vi "Read Dialog Text.vi"(8 "error in (no error)":errorcluster, 11 "Dialog in":refnum<class "Dialog.lvclass">) -> (0 "error out":errorcluster, 2 "Dialog Text":string, 3 "Dialog out":refnum<class "Dialog.lvclass">)   [LabVIEW 2020, in "Dialog Classes.lvlib" / "Dialog.lvclass"]
uses:
  Dialog.lvclass
  Dialog.lvclass/Dialog.ctl
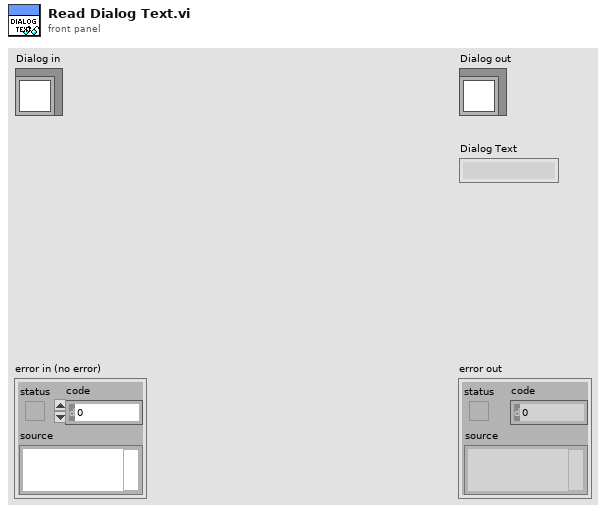
[diagram p1: front panel]
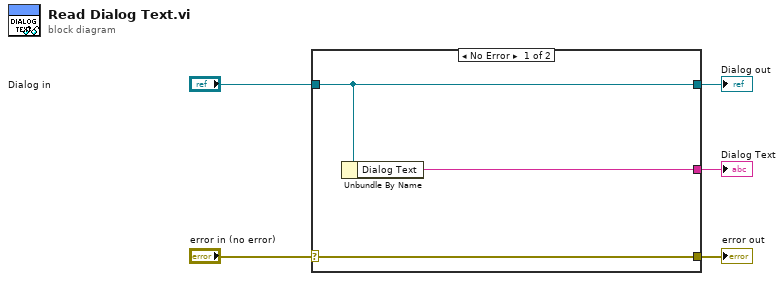
[diagram p0: block diagram]
diagram:
  n1 = case shown="No Error" "error in (no error)" {
    selector: "error in (no error)" -> [w8 w9]
    tunnel: [w8 w9] -> w4
    tunnel: [w7 w10] -> w2
    tunnel: "Dialog in" -> [w7 w10]
    tunnel: [w6 _] -> w1
    frame No Error {
      n2 = Unbundle By Name(w7) -> ("Dialog Text"=w6:string)
    }
    frame Error {
    }
  }
  "error out" <- w4
  "Dialog out" <- w2
  "Dialog Text" <- w1
